vi "Enqueue Controller Element.vi"(7 "Priority Message? (F)":bool, 8 "error in (no error)":errorcluster, 9 "Controller Queue Data":variant, 10 "Controller Queue Message":T1, 11 "Message Queue":refnum<queue>) -> (0 "error out":errorcluster, 3 "dup Message Queue":refnum<queue>)   [LabVIEW 2017]
uses:
  Controller Queue Message Cluster.ctl
  Controller Queue Message.ctl
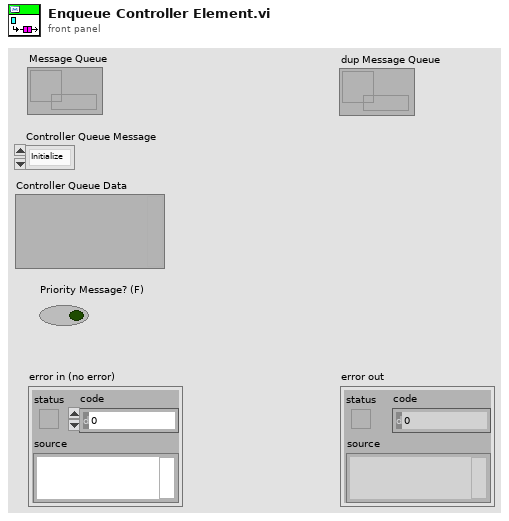
[diagram p1: front panel]
types:
  T1 = typedef "Controller Queue Message.ctl" = enum16{"Initialize", "User Console Update", "Sensor Update", "Wait for First Request", "Start and Move", "Analysis", "Continue Travel", "Stop at Floor", "Open and Close Door Sequence", "Close Door", "No Request Remaining", "Check Time", "Emergency Call", "Terminate Process", "Controller Exit", "Start Exit", "Error Handling"}
  T2 = typedef "Controller Queue Message Cluster.ctl" = cluster{"Controller Queue Message":T1, "Controller Queue Data":variant}
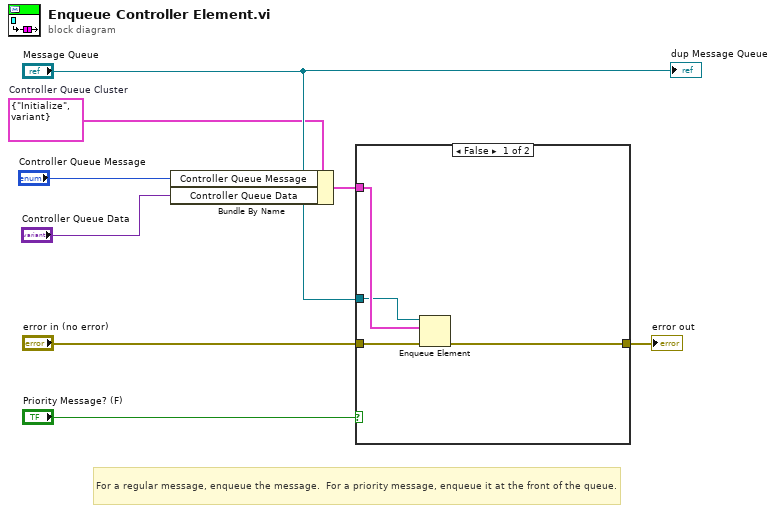
[diagram p0: block diagram]
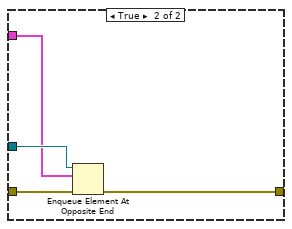
[diagram p2: hidden frame]
diagram:
  w3 = T2 {"Controller Queue Message"=enum."Initialize", "Controller Queue Data"=variant}  # Controller Queue Cluster
  # "For a regular message, enqueue the message.  For a priority message, enqueue it at the front of the queue."
  n1 = Bundle By Name(cluster=w3, "Controller Queue Message"="Controller Queue Message", "Controller Queue Data"="Controller Queue Data") -> (w5:T2)
  n2 = case shown="False" "Priority Message? (F)" {
    tunnel: "error in (no error)" -> [w12 w16]
    tunnel: [w11 w15] -> w6
    tunnel: w5 -> [w10 w13]
    tunnel: "Message Queue" -> [w9 w14]
    frame False {
      n3 = Enqueue Element(queue=w9, element=w10, error in (no error)=w12) -> (error out=w11:errorcluster)  [unwired: 1 in, 2 out]
    }
    frame True {
      n4 = Enqueue Element At Opposite End(queue=w14, element=w13, error in (no error)=w16) -> (error out=w15:errorcluster)  [unwired: 1 in, 2 out]
    }
  }
  "error out" <- w6
  "dup Message Queue" <- "Message Queue"
